vi "Is VI Server Required.vi"(8 "error in (no error)":errorcluster, 11 "Image Assertion in":refnum<class "Image Assertion.lvclass">) -> (0 "error out":errorcluster, 2 "VI Server Required?":bool, 3 "Image Assertion out":refnum<class "Image Assertion.lvclass">)   [LabVIEW 2020, in "MacroAssert.lvlib" / "Image Assertion.lvclass"]
doc: "Outputs whether VI Server is required to perform the given step."
uses:
  Image Assertion.lvclass
  Image Assertion.lvclass/Image Assertion.ctl
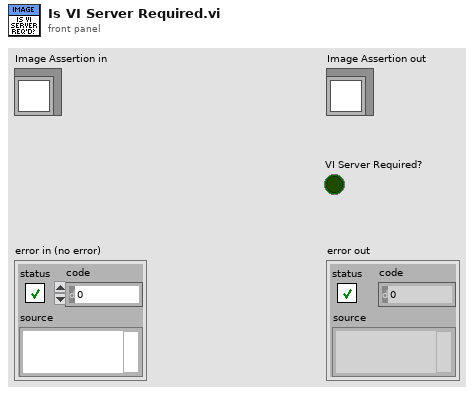
[diagram p1: front panel]
types:
  T1 = typedef "MacroAssert.lvlib/Image Assertion.lvclass/Image Assertion Type.ctl" = enum16{"Control Image", "VI Image", "Window Image", "Cursor Icon"}
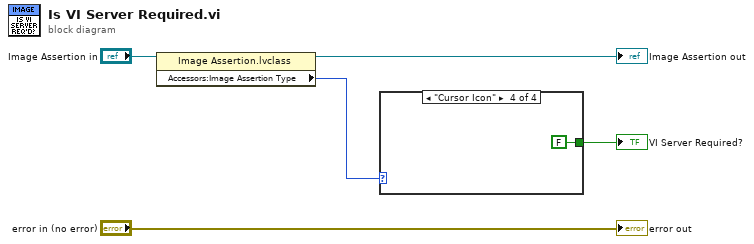
[diagram p0: block diagram]
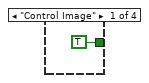
[diagram p2: hidden frame]
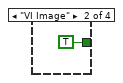
[diagram p3: hidden frame]
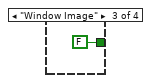
[diagram p4: hidden frame]
diagram:
  n1 = property class="Image Assertion.lvclass"(reference="Image Assertion in") -> (reference out=→"Image Assertion out":refnum<class "Image Assertion.lvclass">, "Accessors:Image Assertion Type"=w5:T1)  [unwired: 1 in, 1 out]
  n2 = case shown="\"Cursor Icon\"" w5 {
    tunnel: [TRUE TRUE FALSE FALSE] -> w3
    frame "Control Image" {
    }
    frame "VI Image" {
    }
    frame "Window Image" {
    }
    frame "Cursor Icon" {
    }
  }
  "VI Server Required?" <- w3
  "error out" <- "error in (no error)"
